vi "Clear HWI.vi"(8 "error in (no error)":errorcluster, 11 "Novatech in":refnum<class "Novatech.lvclass">) -> (0 "error out":errorcluster, 3 "Novatech out":refnum<class "Novatech.lvclass">)   [LabVIEW 2013, in "Novatech.lvclass"]
uses:
  Novatech.lvclass
  Novatech.lvclass/Novatech.ctl
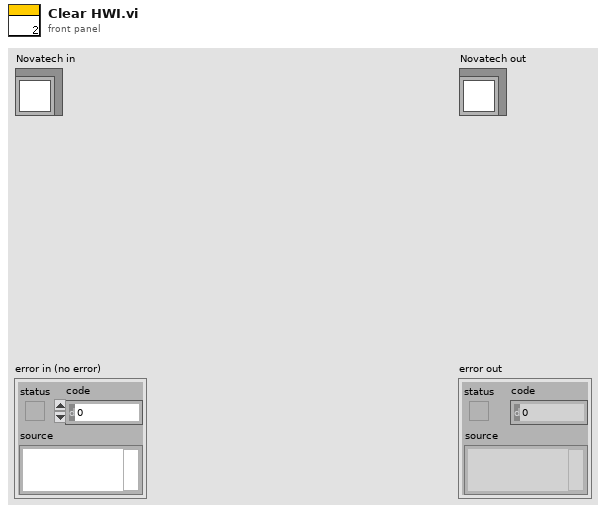
[diagram p1: front panel]
types:
  T1 = cluster{"Freq. [MHz]":dbl[][], "Power [Level]":u16[][], "Phase":u16[][], "2 Freq. [MHz]":dbl, "2 Power [dBm]":u16, "2 phase":u16, "3 Freq. [MHz]":dbl, "3 Power [dBm]":u16, "3 phase":u16}
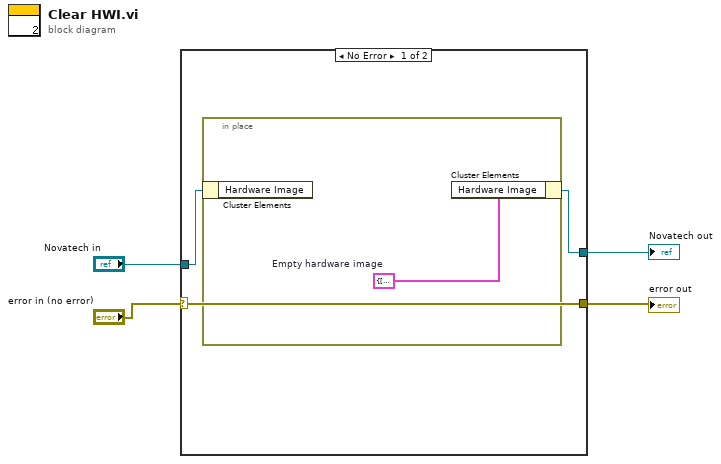
[diagram p0: block diagram]
diagram:
  n1 = case shown="No Error" "error in (no error)" {
    selector: "error in (no error)" -> [w7 w10]
    tunnel: [w7 w10] -> w3
    tunnel: [w6 w9] -> w4
    tunnel: "Novatech in" -> [w5 w9]
    frame No Error {
      n2 = in-place {
        w8 = T1 {"Freq. [MHz]"=[], "Power [Level]"=[], "Phase"=[], "2 Freq. [MHz]"=0.0, "2 Power [dBm]"=0, "2 phase"=0, "3 Freq. [MHz]"=0.0, "3 Power [dBm]"=0, "3 phase"=0}  # Empty hardware image
        n3 = in-place-cluster #1(w5) -> ()  [unwired: 1 out]
        n4 = in-place-cluster #1("Hardware Image"=w8) -> (w6:refnum<class "Novatech.lvclass">)
      }
    }
    frame Error {
    }
  }
  "error out" <- w3
  "Novatech out" <- w4
